vi "Begin.vi"(8 "error in":errorcluster) -> (0 "error out":errorcluster)   [LabVIEW 2019]
doc: "Called before other user functions, this VI is expected to open initial I/O refnums, load in file data, and do all program initialization. Notice that the <B>error out</B> terminal is simply used for data flow. Wiring it to other structures or subVIs ensures that this VI runs first."
uses:
  <vilib>/Rock Robotics/WPI/DriverStation/WPI_DriverStationRobotMode2.ctl
  Typedefs/typedef_enum_Begin_State.ctl
  <vilib>/Rock Robotics/WPI/Joystick/WPI_JoystickDeviceEnum.ctl
  Typedefs/typedef_enum_refnums.ctl
  <vilib>/Rock Robotics/WPI/SafetyOutput/WPI_SafetyOutputConfigMenu.ctl
  <vilib>/Rock Robotics/SystemInterfaces/DIO/FPGA_DIOPWMChannel.ctl
  Robot Global Data.vi
  <vilib>/Rock Robotics/WPI/RobotDrive/WPI_RobotDriveOpen4MotorWithSPARK.vi
  <vilib>/Rock Robotics/WPI/MotorControl/WPI_MotorControlOpen SPARK.vi
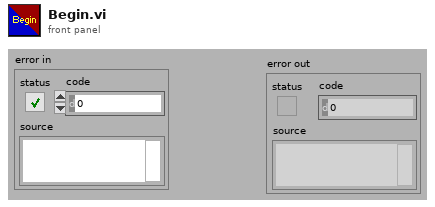
[diagram p1: front panel]
types:
  T1 = typedef "typedef_enum_Begin_State.ctl" = enum16{"Joy_Setup", "Drive_Setup", "Lift_Setup", "Intake_Setup", "Fly_Setup", "Stop"}
  T2 = typedef "WPI_DriverStationRobotMode2.ctl" = enum16{"Autonomous Disabled", "Autonomous Enabled", "Teleop Disabled", "Teleop Enabled", "Disconnected", "Finish", "Test Disabled", "Test Enabled", "Emergency Stopped"}
  T3 = typedef "typedef_enum_refnums.ctl" = enum16{"Joy_L", "Joy_R", "Drive_Motors", "Lift_Motor_M", "Lift_Motor_S", "Intake_Motor", "Fly_Motor_R", "Fly_Motor_L"}
  T4 = typedef "WPI_JoystickDeviceEnum.ctl" = enum16{"USB 0", "USB 1", "USB 2", "USB 3", "USB 4", "USB 5"}
  T5 = typedef "WPI_SafetyOutputConfigMenu.ctl" = enum16{"Enable", "Disable"}
  T6 = enum16{"FollowerType_PercentOutput", "FollowerType_AuxOutput1"}
  T7 = typedef "FPGA_DIOPWMChannel.ctl" = enum8{"PWM 0", "PWM 1", "PWM 2", "PWM 3", "PWM 4", "PWM 5", "PWM 6", "PWM 7", "PWM 8", "PWM 9", "PWM MXP 0", "PWM MXP 1", "PWM MXP 2", "PWM MXP 3", "PWM MXP 4", "PWM MXP 5", "PWM MXP 6", "PWM MXP 7", "PWM MXP 8", "PWM MXP 9", "Invalid"}
  T8 = typedef "WPI_JoystickDevRef.ctl" = cluster{"Device":T4}
  T9 = typedef "WPI_RobotDriveDevRef.ctl" = cluster{"DevStatus":errorcluster, "Motors[]":T10[], "Square Inputs":bool, "Max Output":dbl}
  T10 = typedef "WPI_MotorControlDeviceRef.ctl" = cluster{"DeviceStatus":errorcluster, "Type":T11, "PWM":cluster{"PWM Channel":T7, "DeadBand":T12}, "CAN":cluster{"Device Number":u8, "SetOutput VI Ref":variant, "GetOutput VI Ref":variant, "Enable VI Ref":variant, "Disable VI Ref":variant, "Data":variant}, "Invert":bool, "DIO PWM":cluster{"PWM \"Enable\" Channel":T7, "DIOChannel":T13, "PWM Rate":dbl}}
  T11 = typedef "WPI_MotorControlType.ctl" = enum16{"PWM", "CAN", "DIO PWM"}
  T12 = typedef "WPI_PWMDeadband.ctl" = cluster{"Name":string, "maxPositivePwm":i32, "minPositivePwm":i32, "centerPwm":i32, "maxNegativePwm":i32, "minNegativePwm":i32, "angularRange":u16}
  T13 = typedef "FPGA_DIOChannel.ctl" = enum8{"DIO 0", "DIO 1", "DIO 2", "DIO 3", "DIO 4", "DIO 5", "DIO 6", "DIO 7", "DIO 8", "DIO 9", "DIO MXP 0", "DIO MXP 1", "DIO MXP 2", "DIO MXP 3", "DIO MXP 4", "DIO MXP 5", "DIO MXP 6", "DIO MXP 7", "DIO MXP 8", "DIO MXP 9", "DIO MXP 10", "DIO MXP 11", "DIO MXP 12", "DIO MXP 13", "DIO MXP 14", "DIO MXP 15", "SPI Port CS1", "SPI Port CS2", "SPI Port CS3", "SPI Port MISO", "SPI Port MOSI", "Invalid"}
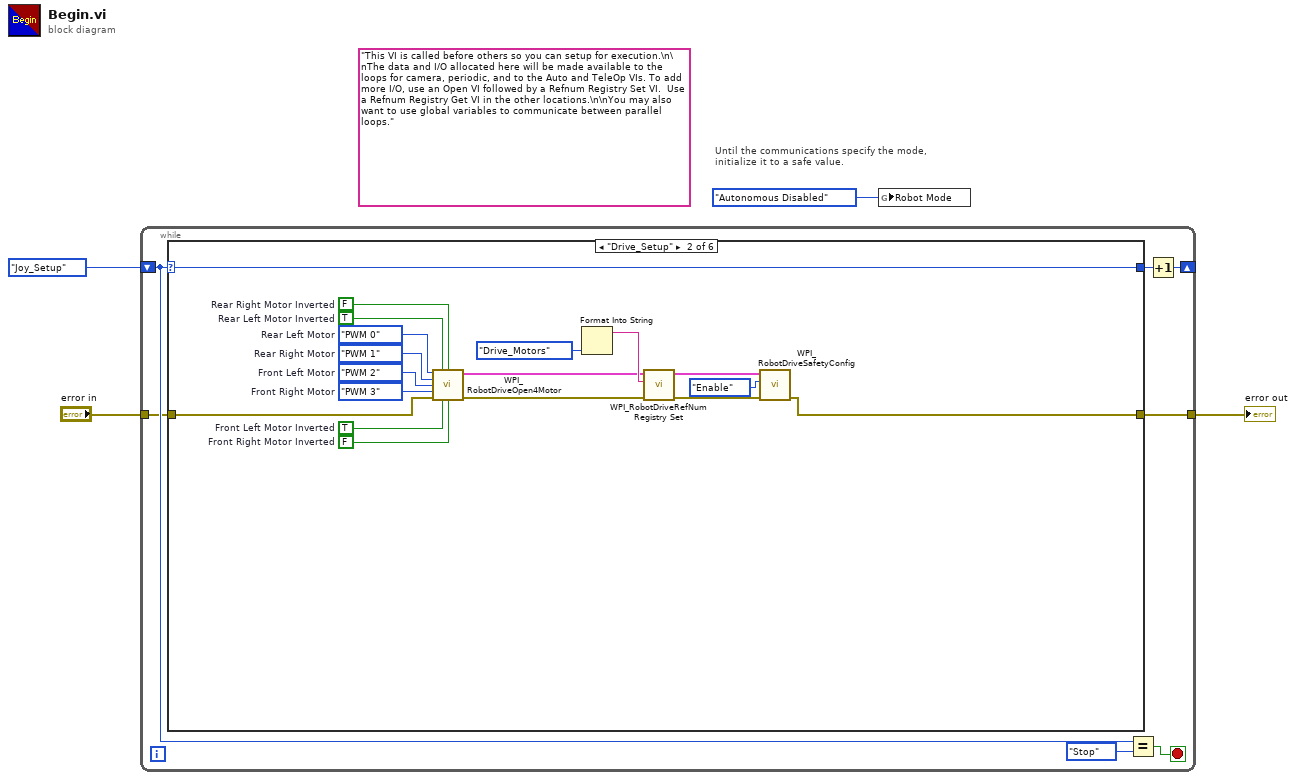
[diagram p0: block diagram]
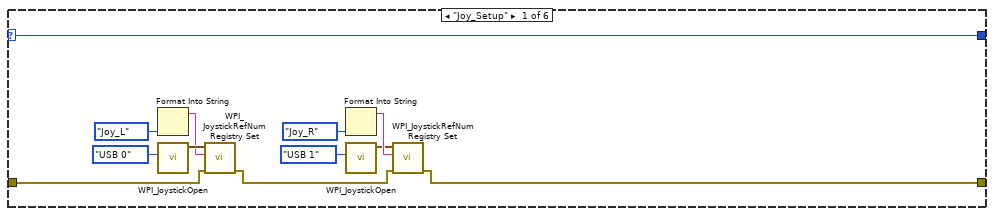
[diagram p2: hidden frame]
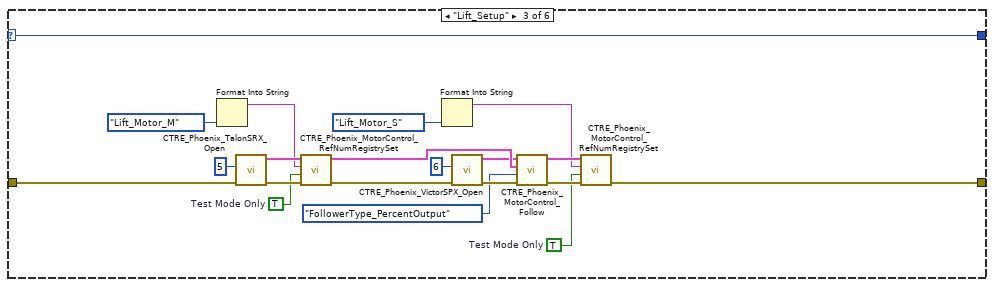
[diagram p3: hidden frame]
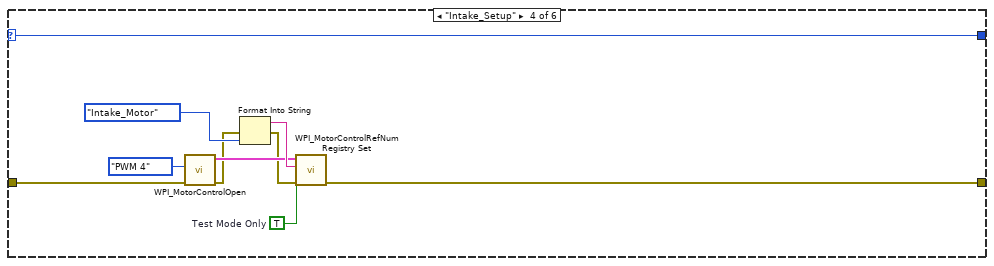
[diagram p4: hidden frame]
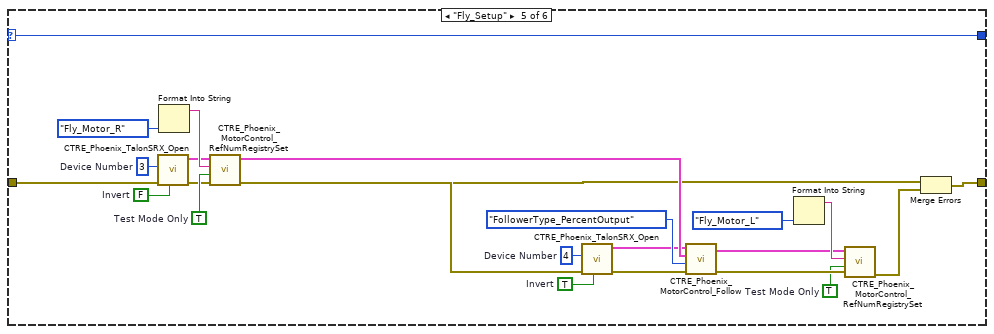
[diagram p5: hidden frame]
diagram:
  (unwired) "This VI is called before others so you can setup for execution.\n\nThe data and I/O allocated here will be made available to the loops for camera, periodic, and to the Auto and TeleOp VIs. To add more I/O, use an Open VI followed by a Refnum Registry Set VI.  Use a Refnum Registry Get VI in the other locations.\n\nYou may also want to use global variables to communicate between parallel loops."
  # "Until the communications specify the mode,\ninitialize it to a safe value."
  n1 = while {
    tunnel: "error in" -> [w8]
    tunnel: [w7] -> w2
    shift-right: [w6] -> _
    shift-left: typedef_enum_Begin_State."Joy_Setup" ("Enum") -> [w11]
    stop <- w9 stop-if-true
    n2 = case shown="\"Drive_Setup\"" w11 {
      selector: w11 -> [w12 w40 w61 w63 w72 w96]
      tunnel: w8 -> [w21 w26 w58 w70 w85 w95]
      tunnel: [w13 w41 w42 w64 w73 w95] -> w7
      tunnel: [w12 w40 w61 w63 w72 w96] -> w5
      frame "Joy_Setup" {
        n3 = Format Into String(typedef_enum_refnums."Joy_L" ("Enum")) -> (resulting string=w19:string)  [unwired: 3 in, 1 out]
        n4 = call <vilib>:"WPI_JoystickOpen.vi"("JoystickDevice"=WPI_JoystickDeviceEnum."USB 0") -> ("JoystickDevRef"=w23:T8)  [unwired: 10 in]
        n5 = call <vilib>:"WPI_JoystickRefNum Registry Set.vi"("error in (no error)"=w21, "refnum name"=w19, "JoystickDevRef"=w23) -> ("error out"=w14:errorcluster)  [unwired: 7 in, 1 out]
        n6 = Format Into String(typedef_enum_refnums."Joy_R" ("Enum")) -> (resulting string=w18:string)  [unwired: 3 in, 1 out]
        n7 = call <vilib>:"WPI_JoystickOpen.vi"("JoystickDevice"=WPI_JoystickDeviceEnum."USB 1") -> ("JoystickDevRef"=w15:T8)  [unwired: 10 in]
        n8 = call <vilib>:"WPI_JoystickRefNum Registry Set.vi"("error in (no error)"=w14, "refnum name"=w18, "JoystickDevRef"=w15) -> ("error out"=w13:errorcluster)  [unwired: 7 in, 1 out]
      }
      frame "Drive_Setup" {
        w27 = FALSE  # Front Right Motor Inverted
        w28 = TRUE  # Front Left Motor Inverted
        w29 = FALSE  # Rear Right Motor Inverted
        w30 = TRUE  # Rear Left Motor Inverted
        w31 = FPGA_DIOPWMChannel."PWM 3"  # Front Right Motor
        w32 = FPGA_DIOPWMChannel."PWM 2"  # Front Left Motor
        w33 = FPGA_DIOPWMChannel."PWM 1"  # Rear Right Motor
        w34 = FPGA_DIOPWMChannel."PWM 0"  # Rear Left Motor
        n9 = call-poly <vilib>:"WPI_RobotDriveOpen4Motor.vi"("Rear Left Motor"=w34, "Rear Left Motor Inverted"=w30, "Rear Right Motor Inverted"=w29, "Rear Right Motor"=w33, "Front Left Motor"=w32, "Front Right Motor"=w31, "error in (no error)"=w26, "Front Left Motor Inverted"=w28, "Front Right Motor Inverted"=w27) -> ("RobotDriveDevRef"=w25:T9, "error out"=w24:errorcluster)  [unwired: 5 in]
        n10 = Format Into String(typedef_enum_refnums."Drive_Motors" ("Enum")) -> (resulting string=w36:string)  [unwired: 3 in, 1 out]
        n11 = call <vilib>:"WPI_RobotDriveRefNum Registry Set.vi"("error in (no error)"=w24, "refnum name"=w36, "RobotDriveDevRef"=w25) -> ("error out"=w35:errorcluster, "RobotDriveDevRef"=w39:T9)  [unwired: 1 in, 6 out]
        n12 = call <vilib>:"WPI_RobotDriveSafetyConfig.vi"("error in (no error)"=w35, "mode"=WPI_SafetyOutputConfigMenu."Enable", "RobotDriveDevRef"=w39) -> ("error out"=w41:errorcluster)  [unwired: 7 in, 1 out]
      }
      frame "Lift_Setup" {
        w43 = TRUE  # Test Mode Only
        w54 = TRUE  # Test Mode Only
        n13 = Format Into String(typedef_enum_refnums."Lift_Motor_M" ("Enum")) -> (resulting string=w56:string)  [unwired: 3 in, 1 out]
        n14 = call <vilib>:"CTRE_Phoenix_TalonSRX_Open.vi"("error in"=w58, "Device Number"=u8 5) -> ("error out"=w55:errorcluster, "CAN Talon SRX Ref"=w57:T10)  [unwired: 8 in]
        n15 = call <vilib>:"CTRE_Phoenix_MotorControl_RefNumRegistrySet.vi"("error in (no error)"=w55, "Test Mode Only"=w54, "refnum name"=w56, "PhoenixMotorControlDevRef"=w57) -> ("error out"=w53:errorcluster, "PhoenixMotorControlDevRef"=w49:T10)  [unwired: 6 in]
        n16 = Format Into String(typedef_enum_refnums."Lift_Motor_S" ("Enum")) -> (resulting string=w44:string)  [unwired: 3 in, 1 out]
        n17 = call <vilib>:"CTRE_Phoenix_VictorSPX_Open.vi"("error in"=w53, "Device Number"=u8 6) -> ("error out"=w50:errorcluster, "CAN Talon SRX Ref"=w48:T10)  [unwired: 8 in]
        n18 = call <vilib>:"CTRE_Phoenix_MotorControl_Follow.vi"("error in (no error)"=w50, "FollowerType"=T6."FollowerType_PercentOutput", "Master Controller to Follow"=w49, "PhoenixMotorControlDevRef"=w48) -> ("error out"=w45:errorcluster, "PhoenixMotorControlDevRef"=w46:T10)  [unwired: 6 in]
        n19 = call <vilib>:"CTRE_Phoenix_MotorControl_RefNumRegistrySet.vi"("error in (no error)"=w45, "Test Mode Only"=w43, "refnum name"=w44, "PhoenixMotorControlDevRef"=w46) -> ("error out"=w42:errorcluster)  [unwired: 6 in, 1 out]
      }
      frame "Intake_Setup" {
        w62 = TRUE  # Test Mode Only
        n20 = call-poly <vilib>:"WPI_MotorControlOpen.vi"("error in (no error)"=w70, "PWM Channel"=FPGA_DIOPWMChannel."PWM 4") -> ("error out"=w66:errorcluster, "MotorControlDeviceRef"=w67:T10)  [unwired: 8 in]
        n21 = Format Into String(error in=w66, typedef_enum_refnums."Intake_Motor" ("Enum")) -> (resulting string=w68:string, error out=w65:errorcluster)  [unwired: 2 in]
        n22 = call <vilib>:"WPI_MotorControlRefNum Registry Set.vi"("error in (no error)"=w65, "Test Mode Only"=w62, "refnum name"=w68, "MotorControlDevRef"=w67) -> ("error out"=w64:errorcluster)  [unwired: 6 in, 1 out]
      }
      frame "Fly_Setup" {
        w77 = TRUE  # Test Mode Only
        w87 = TRUE  # Invert
        w86 = u8 4  # Device Number
        w89 = TRUE  # Test Mode Only
        w93 = FALSE  # Invert
        w94 = u8 3  # Device Number
        n23 = call <vilib>:"CTRE_Phoenix_TalonSRX_Open.vi"("Invert"=w93, "error in"=w85, "Device Number"=w94) -> ("error out"=w88:errorcluster, "CAN Talon SRX Ref"=w90:T10)  [unwired: 7 in]
        n24 = Format Into String(typedef_enum_refnums."Fly_Motor_R" ("Enum")) -> (resulting string=w91:string)  [unwired: 3 in, 1 out]
        n25 = call <vilib>:"CTRE_Phoenix_MotorControl_RefNumRegistrySet.vi"("error in (no error)"=w88, "Test Mode Only"=w89, "refnum name"=w91, "PhoenixMotorControlDevRef"=w90) -> ("error out"=w74:errorcluster, "PhoenixMotorControlDevRef"=w84:T10)  [unwired: 6 in]
        n26 = call <vilib>:"CTRE_Phoenix_TalonSRX_Open.vi"("Invert"=w87, "error in"=w85, "Device Number"=w86) -> ("error out"=w82:errorcluster, "CAN Talon SRX Ref"=w81:T10)  [unwired: 7 in]
        n27 = call <vilib>:"CTRE_Phoenix_MotorControl_Follow.vi"("error in (no error)"=w82, "FollowerType"=T6."FollowerType_PercentOutput", "Master Controller to Follow"=w84, "PhoenixMotorControlDevRef"=w81) -> ("error out"=w78:errorcluster, "PhoenixMotorControlDevRef"=w79:T10)  [unwired: 6 in]
        n28 = Format Into String(typedef_enum_refnums."Fly_Motor_L" ("Enum")) -> (resulting string=w80:string)  [unwired: 3 in, 1 out]
        n29 = call <vilib>:"CTRE_Phoenix_MotorControl_RefNumRegistrySet.vi"("error in (no error)"=w78, "Test Mode Only"=w77, "refnum name"=w80, "PhoenixMotorControlDevRef"=w79) -> ("error out"=w75:errorcluster)  [unwired: 6 in, 1 out]
        n30 = Merge Errors(w74, w75) -> (w73:errorcluster)
      }
      frame "Stop" {
      }
    }
    n31 = Equal?(x=w11, y=typedef_enum_Begin_State."Stop") -> (x = y?=w9:bool)
    n32 = Increment(x=w5) -> (x+1=w6:T1)
  }
  "error out" <- w2
  n33 = global write "Robot Global Data.vi" "Robot Mode"(WPI_DriverStationRobotMode2."Autonomous Disabled" ("Robot Mode")) -> ()
